vi "Write and Read.vi"(6 "Delay Before Read (ms)":i32, 7 "Write & Read":bool, 8 "error in (no error)":errorcluster, 9 "Command":string, 10 "VISA Refnum in":refnum<visa-resource-name>, 11 "ESM303 in":refnum<class "ESM303.lvclass">) -> (0 "error out":errorcluster, 1 "Response":string, 3 "ESM303 out":refnum<class "ESM303.lvclass">)   [LabVIEW 2018, in "ESM303.lvlib" / "ESM303.lvclass"]
uses:
  ESM303.lvclass
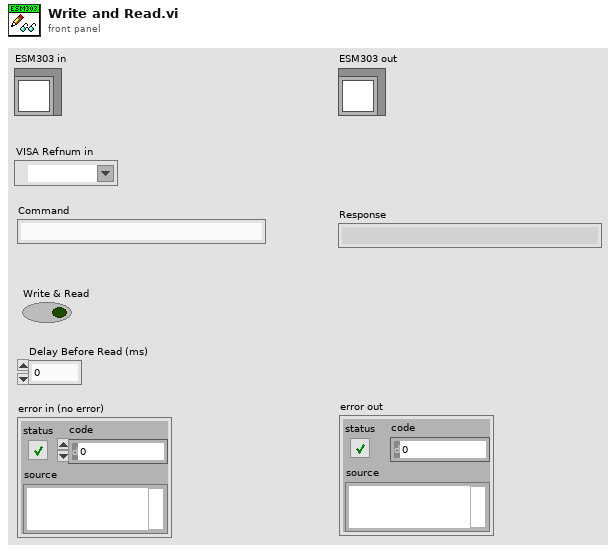
[diagram p1: front panel]
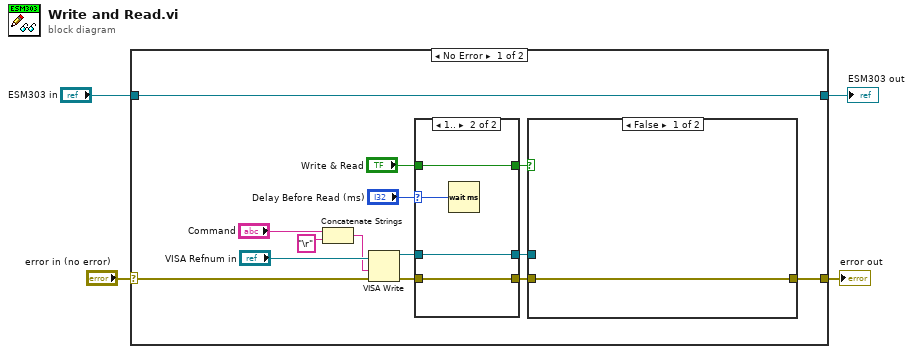
[diagram p0: block diagram]
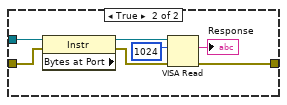
[diagram p3: hidden frame]
diagram:
  n1 = case shown="No Error" "error in (no error)" {
    selector: "error in (no error)" -> [w6 w35]
    tunnel: [w13 w35] -> w4
    tunnel: [w5 w34] -> w2
    tunnel: "ESM303 in" -> [w5 w34]
    frame No Error {
      n2 = Concatenate Strings("Command", "\r" ("string")) -> (w11:string)
      n3 = VISA Write(VISA resource name="VISA Refnum in", write buffer=w11, error in (no error)=w6) -> (VISA resource name out=w18:refnum<visa-resource-name>, error out=w16:errorcluster)  [unwired: 1 out]
      n4 = case shown="1.." "Delay Before Read (ms)" {
        selector: "Delay Before Read (ms)" -> [_ w25]
        tunnel: [w21 w23] -> w15
        tunnel: w16 -> [w21 w23]
        tunnel: [w20 w24] -> w17
        tunnel: w18 -> [w20 w24]
        tunnel: [w19 w22] -> w8
        tunnel: "Write & Read" -> [w19 w22]
        frame 0, Default {
        }
        frame 1.. {
          n5 = Wait (ms)(milliseconds to wait=w25) -> ()  [unwired: 1 out]
        }
      }
      n6 = case shown="False" w8 {
        tunnel: w17 -> [_ w33]
        tunnel: w15 -> [w26 w32]
        tunnel: [w26 w28] -> w13
        frame False {
        }
        frame True {
          n7 = property class="Instr" props=["Bytes at Port"](reference=w33, error in=w32) -> (reference out=w31:refnum<visa-resource-name>, error out=w30:errorcluster)  [unwired: 1 out]
          n8 = VISA Read(VISA resource name=w31, byte count=u32 1024, error in (no error)=w30) -> (read buffer=→"Response":string, error out=w28:errorcluster)  [unwired: 2 out]
        }
      }
    }
    frame Error {
    }
  }
  "error out" <- w4
  "ESM303 out" <- w2
